vi "Login.vi"() -> ()   [LabVIEW 2015]
uses:
  <vilib>/Utility/config.llb/Read Key (String).vi
  <vilib>/Utility/config.llb/NI_LVConfig.lvlib
panel:
  in  "Username":string
  in  "Password":string
  out "Boolean":bool
  in  "stop":bool
  in  "OK Button":bool
  out "error out":errorcluster
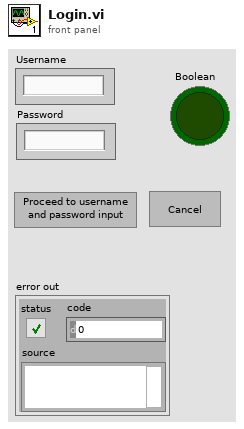
[diagram p1: front panel]
types:
  T1 = typedef "NI_LVConfig.lvlib/Config Data RefNum.ctl" = refnum<k1>
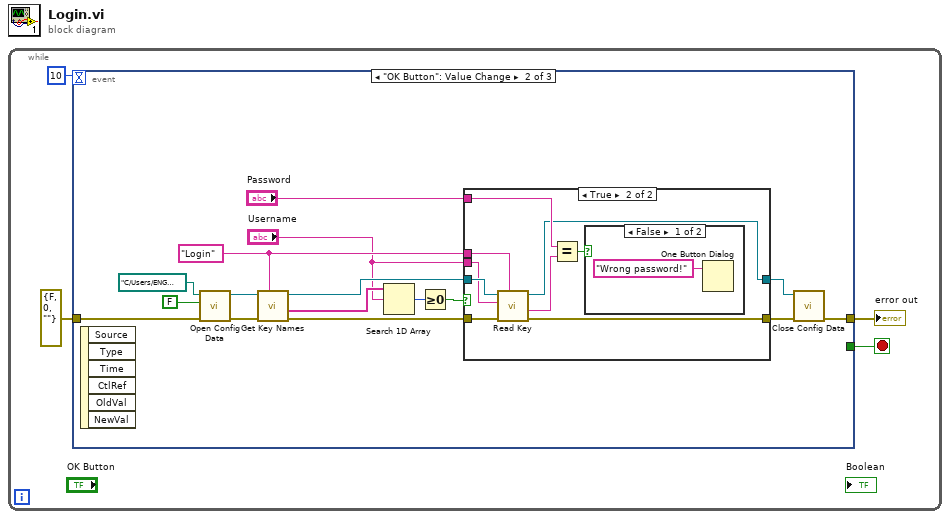
[diagram p0: block diagram]
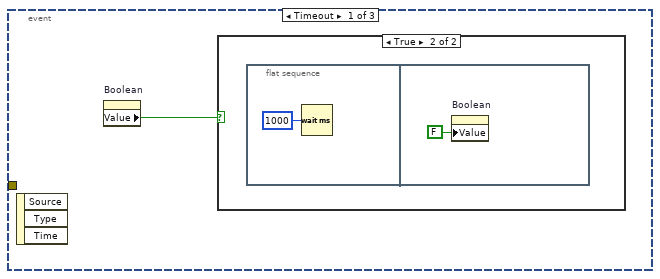
[diagram p2: hidden frame]
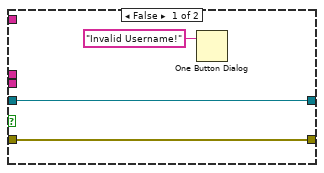
[diagram p4: hidden frame]
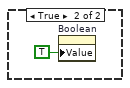
[diagram p5: hidden frame]
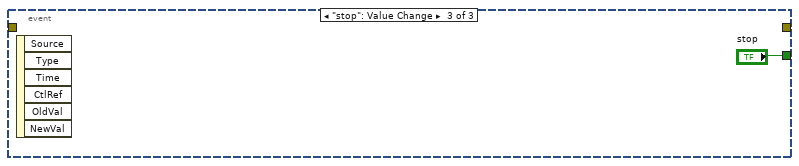
[diagram p6: hidden frame]
diagram:
  n1 = while {
    stop <- w2 stop-if-true
    n2 = event shown="[1] \"OK Button\": Value Change" {
      selector: _ -> [_ _ _]
      dyn-events: _ -> [_ _ _]
      timeout: 10 -> [_ _ _]
      tunnel: errorcluster {"status"=FALSE, "code"=0, "source"=""} ("error in (no error)") -> [_ w23 _]
      tunnel: [_ w10 _] -> w3
      tunnel: [_ _ "stop"] -> w2
      event Timeout {
        n3 = event-data() -> ()  [unwired: 1 in, 3 out]
        n4 = property on="Boolean" class="Bool (strict)"() -> ("Value"=w5:bool)  [unwired: 2 in, 2 out]
        n5 = case shown="True" w5 {
          frame False {
          }
          frame True {
            n6 = flat-sequence {
              frame #0 {
                n7 = Wait (ms)(milliseconds to wait=u32 1000) -> ()  [unwired: 1 out]
              }
              frame #1 {
                n8 = property on="Boolean" class="Bool (strict)"("Value"=FALSE ("Boolean")) -> ()  [unwired: 2 in, 2 out]
              }
            }
          }
        }
      }
      event "OK Button": Value Change {
        w14 = "Login" ("section")
        n9 = event-data() -> ()  [unwired: 1 in, 6 out]
        n10 = call <vilib>:"Open Config Data.vi"("error in (no error)"=w23, "create file if necessary (T)"=FALSE, "configuration file path"=path "C:/Users/ENG User/Downloads/NamesAndPasswords.txt") -> ("error out"=w20:errorcluster, "refnum"=w19:T1)  [unwired: 6 in, 1 out]
        n11 = call <vilib>:"Get Key Names.vi"("section"=w14, "error in (no error)"=w20, "refnum"=w19) -> ("error out"=w13:errorcluster, "key names"=w18:string[], "refnum out"=w15:T1)  [unwired: 5 in, 1 out]
        n12 = Search 1D Array(1D array=w18, element="Username") -> (index of element=w17:i32)  [unwired: 1 in]
        n13 = Greater Or Equal To 0?(x=w17) -> (x >= 0?=w16:bool)
        n14 = case shown="True" w16 {
          tunnel: w15 -> [w25 w35]
          tunnel: w14 -> [_ w34]
          tunnel: "Username" -> [_ w33]
          tunnel: w13 -> [w24 w32]
          tunnel: "Password" -> [_ w30]
          tunnel: [w24 w27] -> w12
          tunnel: [w25 w28] -> w11
          frame False {
            n15 = One Button Dialog(message="Invalid Username!") -> ()  [unwired: 1 in, 1 out]
          }
          frame True {
            n16 = call-poly <vilib>:"Read Key.vi"("section"=w34, "error in (no error)"=w32, "key"=w33, "refnum"=w35) -> ("error out"=w27:errorcluster, "value"=w31:string, "refnum out"=w28:T1)  [unwired: 4 in, 1 out]
            n17 = Equal?(x=w30, y=w31) -> (x = y?=w29:bool)
            n18 = case shown="False" w29 {
              frame False {
                n19 = One Button Dialog(message="Wrong password!") -> ()  [unwired: 1 in, 1 out]
              }
              frame True {
                n20 = property on="Boolean" class="Bool (strict)"("Value"=TRUE ("Boolean")) -> ()  [unwired: 2 in, 2 out]
              }
            }
          }
        }
        n21 = call <vilib>:"Close Config Data.vi"("error in (no error)"=w12, "refnum"=w11) -> ("error out"=w10:errorcluster)  [unwired: 8 in, 1 out]
      }
      event "stop": Value Change {
        n22 = event-data() -> ()  [unwired: 1 in, 6 out]
      }
    }
    "error out" <- w3
  }
